vi "LS_DAQ_Cluster_Host.vi"() -> ()   [LabVIEW 2020]
panel:
  out "Temperature [°C]":dbl format="%#_3g"
  out "Pulse count":dbl
  out "Frequency [Hz]":dbl
  out "Waveform Chart":cluster{"Reading":dbl, "Reading":dbl}(graph)
  in  "Log data":bool
  in  "stop":bool
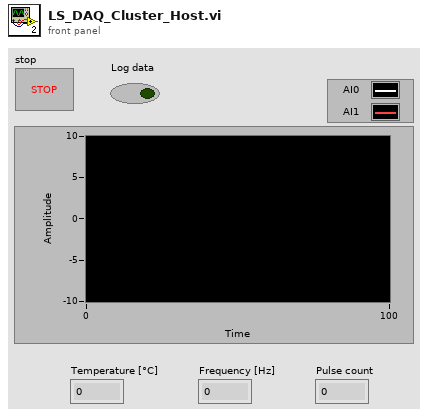
[diagram p1: front panel]
types:
  T1 = enum16{"open", "replace", "create", "open or create", "replace or create", "replace or create with confirmation"}
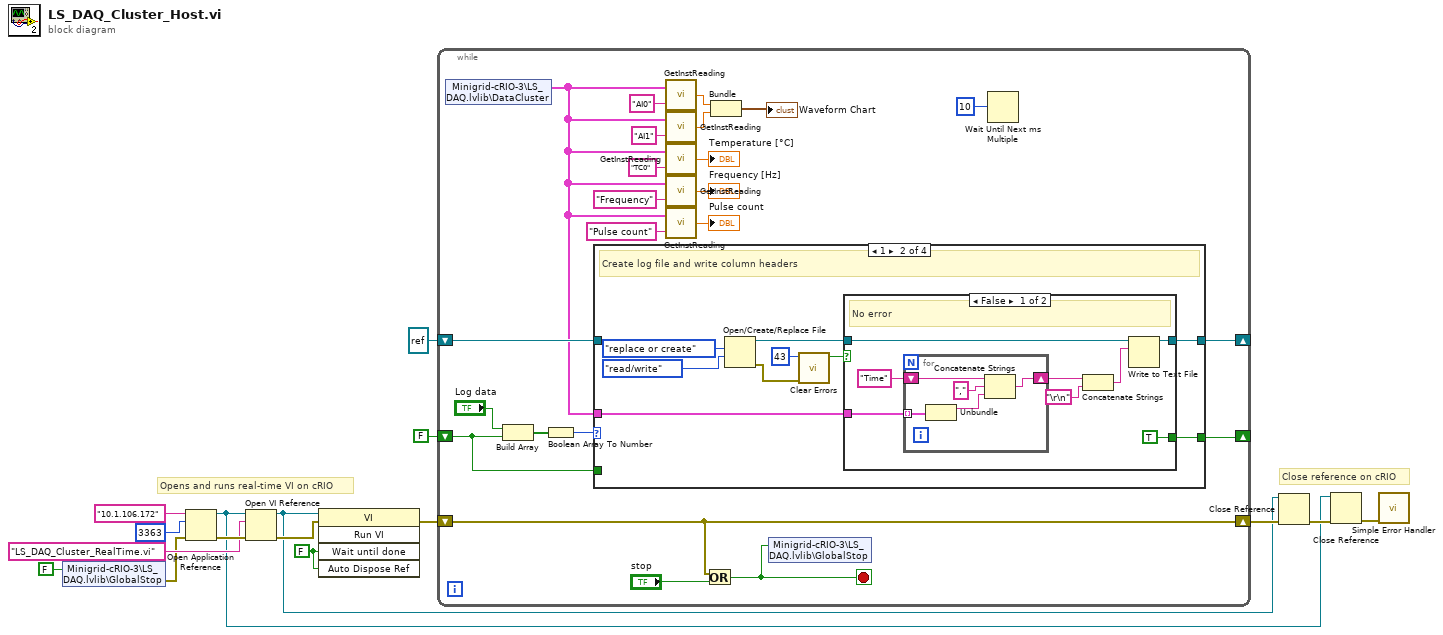
[diagram p0: block diagram]
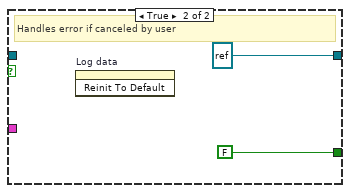
[diagram p3: hidden frame]
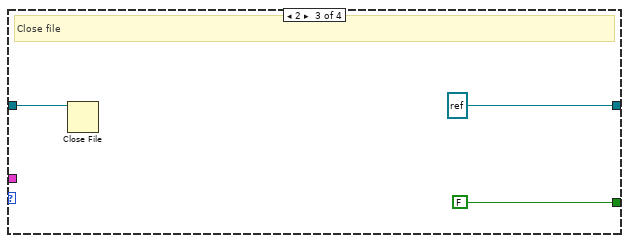
[diagram p4: hidden frame]
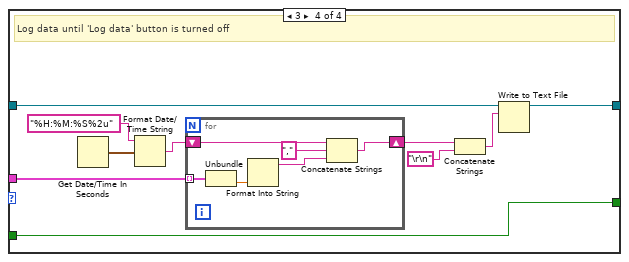
[diagram p5: hidden frame]
diagram:
  w1 = FALSE ("Wait Until Done")
  # "Close reference on cRIO"
  # "Opens and runs real-time VI on cRIO"
  n1 = shared-variable "Minigrid-cRIO-3\\LS_DAQ.lvlib\\GlobalStop"(FALSE ("GlobalStop")) -> (error out=w2:errorcluster)  [unwired: 1 in]
  n2 = Open Application Reference(8:w2, 10:u16 3363 ("port number or service name (3363)"), 11:"10.1.106.172" ("machine name (\"\":  open local reference)")) -> (0:w14:errorcluster, 3:w7:refnum<vi>)  [unwired: 1 in]
  n3 = Open VI Reference(application reference (local)=w7, vi path="LS_DAQ_Cluster_RealTime.vi" ("machine name (\"\":  open local reference)"), error in (no error)=w14) -> (vi reference=w9:refnum<vi>, error out=w13:errorcluster)  [unwired: 3 in]
  n4 = invoke class="VI" method="Run VI"(reference=w9, error in=w13, "Wait until done"=w1, "Auto Dispose Ref"=w1) -> (error out=w12:errorcluster)  [unwired: 1 in, 4 out]
  n5 = while {
    shift-right: [w38] -> w10
    shift-left: w12 -> [w38]
    shift-right: [w32] -> _
    shift-left: FALSE -> [w31]
    shift-right: [w33] -> _
    shift-left: refnum<file> refnum ("refnum out") -> [w30]
    stop <- w37 stop-if-true
    n6 = shared-variable "Minigrid-cRIO-3\\LS_DAQ.lvlib\\DataCluster"() -> (w19:cluster{"Inst. #":string, "Value":dbl}[])  [unwired: 1 in, 1 out]
    n7 = Build Array("Log data", w31) -> (w34:bool[])
    n8 = Boolean Array To Number(Boolean array=w34) -> (number=w36:u32)
    n9 = case shown="1" w36 {
      tunnel: [w40 w47 refnum<file> refnum ("refnum out") w74] -> w33
      tunnel: [w41 w46 FALSE w73] -> w32
      tunnel: w31 -> [w41 _ _ w73]
      tunnel: w30 -> [w40 _ w68 w78]
      tunnel: w19 -> [_ w42 _ w69]
      frame 0, Default {
      }
      frame 1 {
        # "Create log file and write column headers"
        n10 = Open/Create/Replace File(operation (0:open)=T1."replace or create", access (0:read/write)=enum16{"read/write", "read-only", "write-only"}."read/write") -> (refnum out=w48:refnum<file>, error out=w45:errorcluster)  [unwired: 4 in, 1 out]
        n11 = call <vilib>:"Clear Errors.vi"("error in (no error)"=w45, "specific error code to clear (0: all)"=43) -> ("specific error cleared?"=w43:bool)  [unwired: 4 in, 1 out]
        n12 = case shown="False" w43 {
          tunnel: w48 -> [w58 _]
          tunnel: [w57 refnum<file> refnum ("refnum out")] -> w47
          tunnel: [TRUE FALSE] -> w46
          tunnel: w42 -> [w54 _]
          frame False {
            # "No error"
            n13 = for {
              shift-right: [w63] -> w53
              shift-left: "Time" ("string") -> [w62]
              tunnel: w54 -> [w60] mode=indexing
              n14 = Unbundle(w60) -> ("Inst. #"=w59:string)  [unwired: 1 out]
              n15 = Concatenate Strings(w62, "," ("string"), w59) -> (w63:string)
            }
            n16 = Concatenate Strings(w53, "\r\n") -> (w51:string)
            n17 = Write to Text File(file (use dialog)=w58, text=w51) -> (refnum out=w57:refnum<file>)  [unwired: 2 in, 2 out]
          }
          frame True {
            # "Handles error if canceled by user"
            n18 = invoke on="Log data" class="Bool (strict)" method="Reinit To Default"() -> ()  [unwired: 3 in, 3 out]
          }
        }
      }
      frame 2 {
        # "Close file"
        n19 = Close File(refnum=w68) -> ()  [unwired: 1 in, 2 out]
      }
      frame 3 {
        # "Log data until 'Log data' button is turned off"
        n20 = Get Date/Time In Seconds() -> (seconds since 1Jan1904=w72:timestamp)
        n21 = Format Date/Time String(time format string (%c)="%H:%M:%S%2u", seconds (now)=w72) -> (date/time string=w70:string)  [unwired: 1 in]
        n22 = for {
          shift-right: [w81] -> w77
          shift-left: w70 -> [w84]
          tunnel: w69 -> [w80] mode=indexing
          n23 = Unbundle(w80) -> ("Value"=w79:dbl)  [unwired: 1 out]
          n24 = Format Into String(w79) -> (resulting string=w82:string)  [unwired: 3 in, 1 out]
          n25 = Concatenate Strings(w84, "," ("string"), w82) -> (w81:string)
        }
        n26 = Concatenate Strings(w77, "\r\n") -> (w75:string)
        n27 = Write to Text File(file (use dialog)=w78, text=w75) -> (refnum out=w74:refnum<file>)  [unwired: 2 in, 2 out]
      }
    }
    n28 = call "GetInstReading.vi"("Inst number"="AI0", "Array"=w19) -> ("Reading"=w27:dbl)
    n29 = call "GetInstReading.vi"("Inst number"="AI1", "Array"=w19) -> ("Reading"=w26:dbl)
    n30 = call "GetInstReading.vi"("Inst number"="TC0", "Array"=w19) -> ("Reading"=→"Temperature [°C]":dbl)
    n31 = call "GetInstReading.vi"("Inst number"="Frequency", "Array"=w19) -> ("Reading"=→"Frequency [Hz]":dbl)
    n32 = call "GetInstReading.vi"("Inst number"="Pulse count", "Array"=w19) -> ("Reading"=→"Pulse count":dbl)
    n33 = Or(x=w38, y="stop") -> (x .or. y?=w37:bool)
    n34 = Bundle("Reading"=w27, "Reading"=w26) -> (→"Waveform Chart":cluster{"Reading":dbl, "Reading":dbl})  [unwired: 1 in]
    n35 = shared-variable "Minigrid-cRIO-3\\LS_DAQ.lvlib\\GlobalStop"(w37) -> ()  [unwired: 1 in, 1 out]
    n36 = Wait Until Next ms Multiple(millisecond multiple=u32 10 ("milliseconds to wait")) -> ()  [unwired: 1 out]
  }
  n37 = Close Reference(reference=w9, error in (no error)=w10) -> (error out=w8:errorcluster)
  n38 = Close Reference(reference=w7, error in (no error)=w8) -> (error out=w6:errorcluster)
  n39 = call <vilib>:"Simple Error Handler.vi"("error in (no error)"=w6) -> ()  [unwired: 4 in, 5 out]
